vi "Error-Not Error.vi"(3 "error in (no error)":errorcluster) -> (1 "not error":bool)   [LabVIEW 2020]
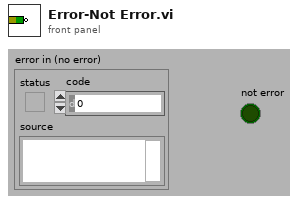
[diagram p1: front panel]
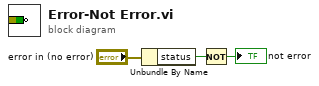
[diagram p0: block diagram]
diagram:
  n1 = Unbundle By Name("error in (no error)") -> ("status"=w2:bool)
  n2 = Not(x=w2) -> (.not. x?=→"not error":bool)
